vi "flow-builder.nutrition-sample.vi"(7 "Proc Name":string, 10 "Unit Index":i32) -> (0 "error out":errorcluster, 1 "status":string, 2 "Nutrition Will Dose?":bool, 3 "intructions out":variant[](array[variant]), 4 "Unit Enable?":bool)   [LabVIEW 2024]
uses:
  controls/UiStepBuilder.ctl
  controls/type.step-builder.ctl
  <vilib>/Utility/error.llb/Trim Whitespace.vi
  build.flowToVarient.vi
  <vilib>/Utility/error.llb/Trim Whitespace One-Sided.vi
  Polymorphics/variantCtrl.polymorphic.vi
  Polymorphics/variantCtrlStepFunction.vi
  Polymorphics/variantCtrlSetpoint.vi
  Polymorphics/variantCtrlString.vi
  proc.util.enumToStrStepVar.vi
  Polymorphics/variantCtrlNumber.vi
  util.DelimitedStringToArray.vi
  proc.util.validateParamExist.vi
  globals/globals-engine.vi
  build.elementToParamString.vi
  util.error.create.vi
  Polymorphics/variantCtrlStepPointer.vi
  Polymorphics/variantCtrlStepUserMessage.vi
  Polymorphics/variantCtrlStepPath.vi
panel:
  out "water Will Dose?":bool
  out "Flow":T1[](array[typedef])
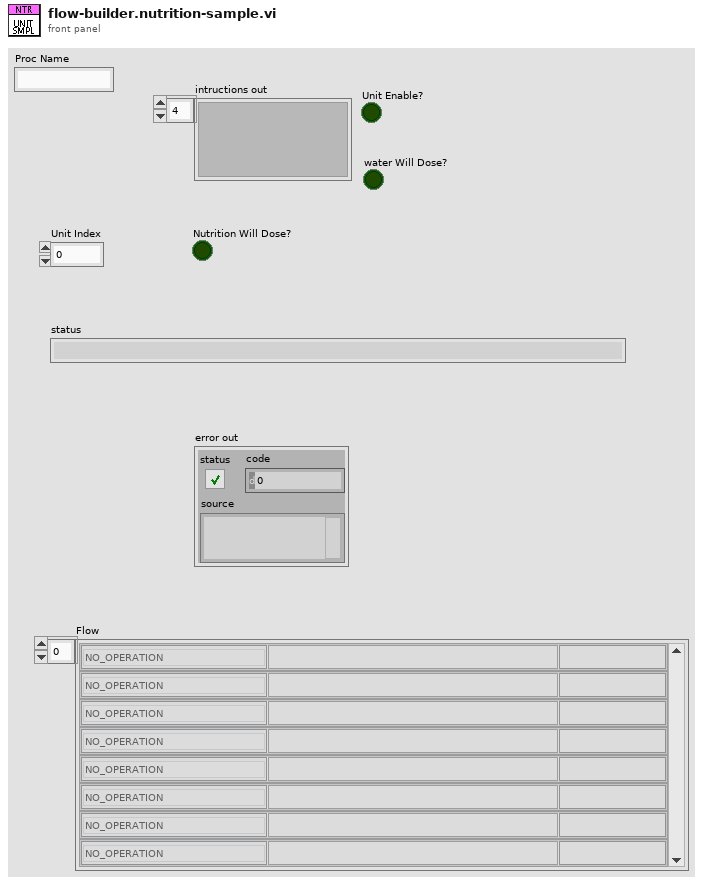
[diagram p1: front panel]
types:
  T1 = typedef "UiStepBuilder.ctl" = cluster{"Step Function":T2, "ParamString":string, "Step Label":string}
  T2 = typedef "type.step-builder.ctl" = enum16{"NO_OPERATION", "DELAY-JUMP", "DELAY", "JUMP", "COMPLETE", "SCHEDULER", "IRR-CHECK", "UNIT-CHECK", "UNIT-SAMPLE", "UNIT-DOSE", "LOG-REPORT", "LOG-MESSAGE", "IO-READ", "IO-READ-MANY", "IO-WRITE", "IO-COMPARE-OUT", "IO-COMPARE-IN", "PROC-START", "PROC-STOP", "PROC-LOAD", "PROC-IS-COMPLETED", "RECORD-MOVE", "GET-RH", "GET-UV", "GET-WD", "GET-WS", "OCS-CHECK", "OCS-RECORD"}
  T3 = typedef "UiNutritionPanel.ctl" = cluster{"Main":cluster{"Enable":bool, "WashTimes":cluster{"In":dbl, "Out":dbl}, "DailyActivityHours":cluster{"Begin Time":T4, "End Time":T4}[]}, "Water Dosing":cluster{"Water Dose":dbl, "Water Limit":dbl}, "EC Ranges":cluster{"H Alarm":dbl, "L Alarm":dbl, "Low":dbl}, "EC Dosing":cluster{"ALFA1 Dose":dbl, "ALFA1 Limit":dbl, "BETA1 Dose":dbl, "BETA1 Limit":dbl, "ALFA2 Dose":dbl, "ALFA2 Limit":dbl, "BETA2 Dose":dbl, "BETA2 Limit":dbl}, "PH Ranges":cluster{"H Alarm":dbl, "L Alarm":dbl, "High":dbl, "Low":dbl}, "PH Dosing":cluster{"ACID Dose":dbl, "ACID Limit":dbl, "BASE Dose":dbl, "BASE Limit":dbl}, "ORP Ranges":cluster{"H Alarm":dbl, "L Alarm":dbl, "Low":dbl}, "ORP Dosing":cluster{"MIX Dose":dbl, "MIX Limit":dbl}}
  T4 = typedef "UiScheduleTimestamp.ctl" = timestamp
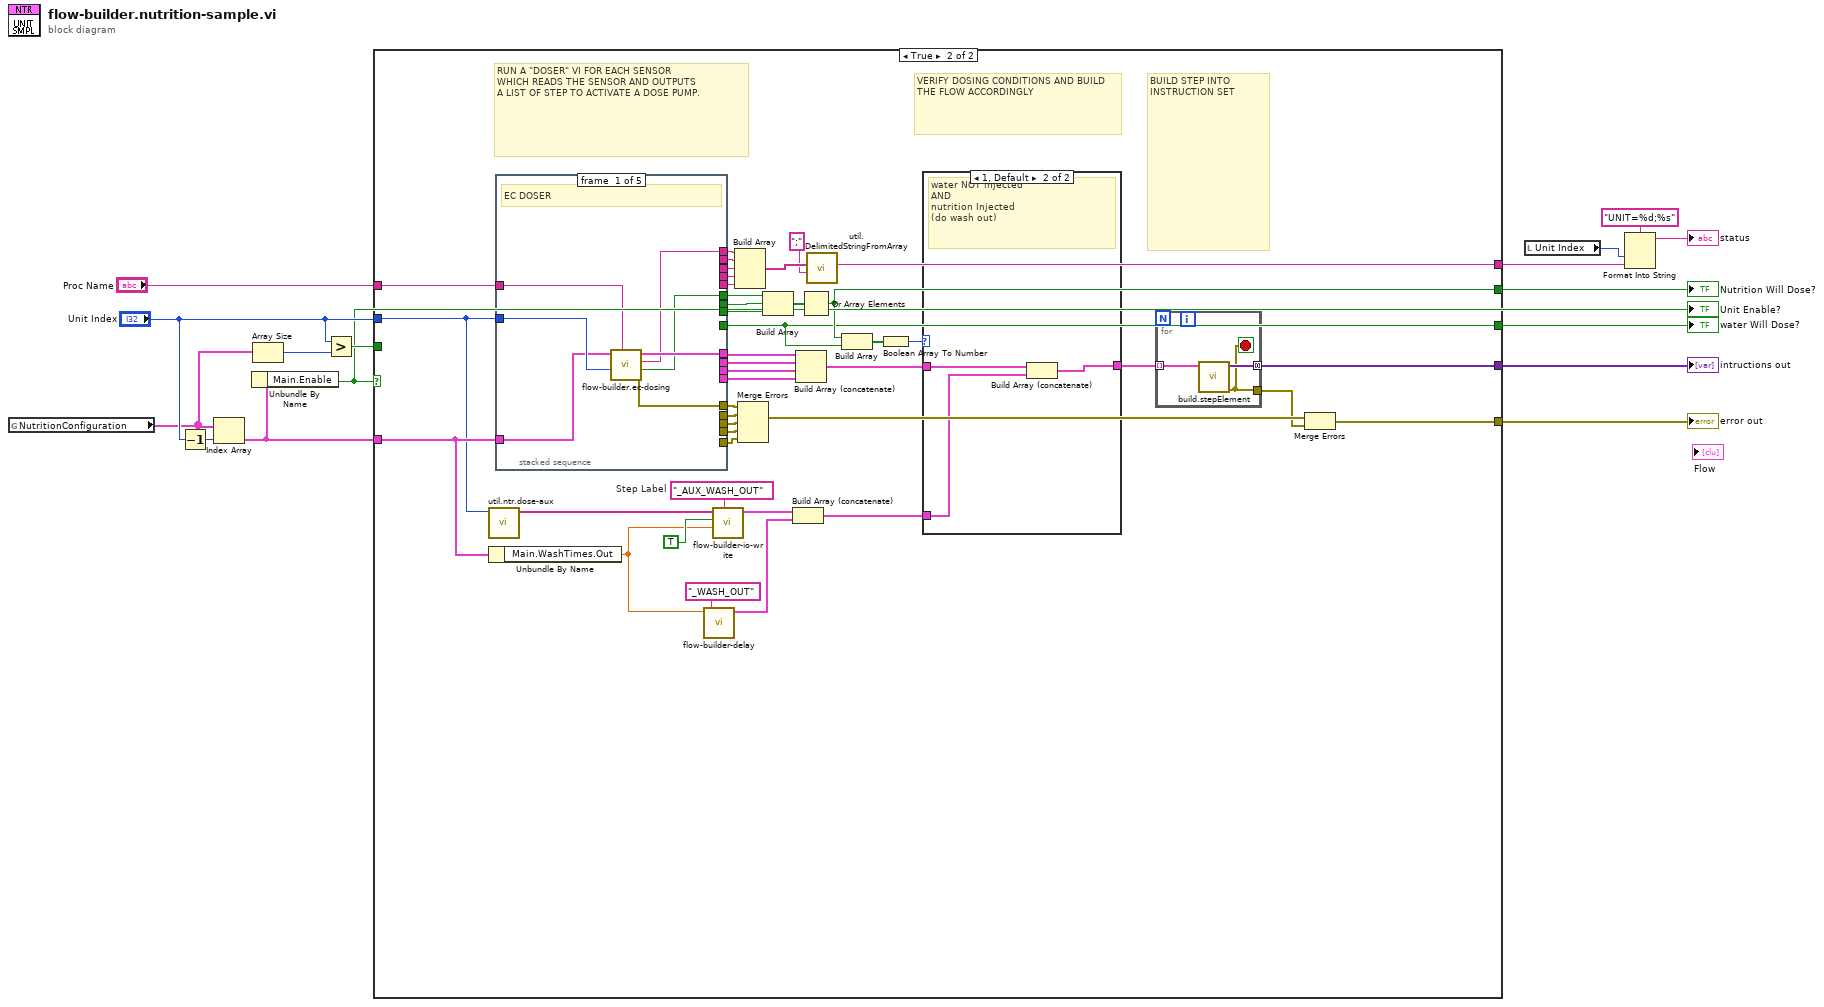
[diagram p0: block diagram]
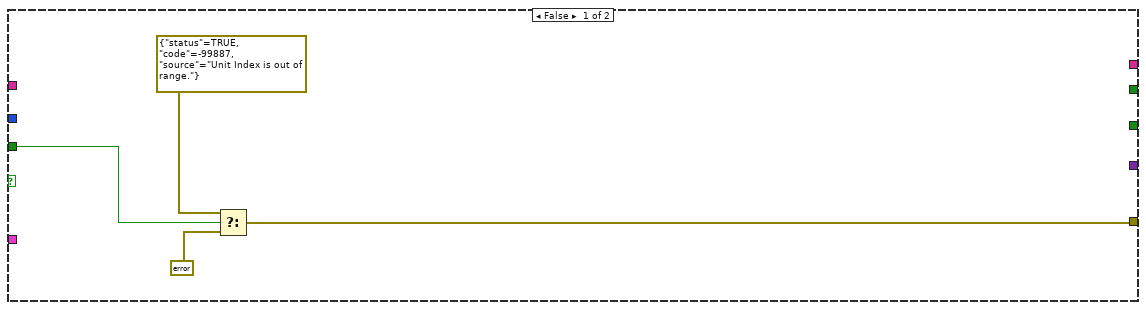
[diagram p2: hidden frame]
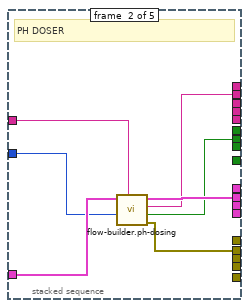
[diagram p4: hidden frame]
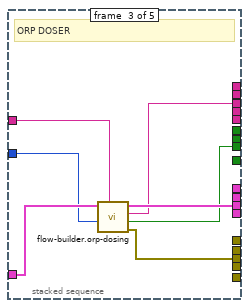
[diagram p5: hidden frame]
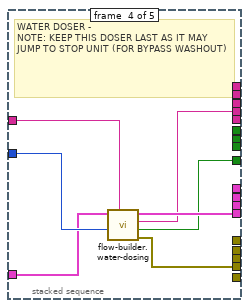
[diagram p6: hidden frame]
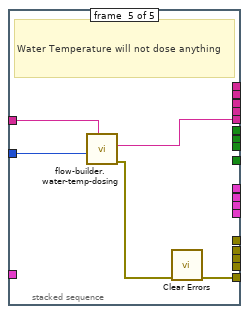
[diagram p7: hidden frame]
diagram:
  n1 = global read "globals-engine.vi" "NutritionConfiguration"() -> (w1:T3[])
  n2 = Decrement(x="Unit Index") -> (x-1=w14:i32)
  n3 = Index Array(array=w1, index=w14) -> (element=w13:T3)
  n4 = Unbundle By Name(w13) -> ("Main.Enable"=w4:bool)
  "Unit Enable?" <- w4
  n5 = Array Size(array=w1) -> (size(s)=w12:i32)
  n6 = Greater?(x="Unit Index", y=w12) -> (0:w11:bool)
  n7 = case shown="True" w4 {
    tunnel: [_ w35] -> w5
    tunnel: [_ w62] -> w16
    tunnel: [w18 w53] -> w15
    tunnel: "Unit Index" -> [_ w32]
    tunnel: w13 -> [_ w34]
    tunnel: w11 -> [w17 _]
    tunnel: [_ w49] -> w10
    tunnel: "Proc Name" -> [_ w33]
    tunnel: [_ w23] -> w3
    frame False {
      n8 = Select(t=errorcluster {"status"=TRUE, "code"=-99887, "source"="Unit Index is out of range."} ("error IO"), s=w17, f=errorcluster {"status"=FALSE, "code"=0, "source"=""} ("error IO")) -> (s? t:f=w18:errorcluster)
    }
    frame True {
      w26 = "_AUX_WASH_OUT"  # Step Label
      # "BUILD STEP INTO INSTRUCTION SET"
      # "VERIFY DOSING CONDITIONS AND BUILD THE FLOW ACCORDINGLY"
      # "RUN A \"DOSER\" VI FOR EACH SENSOR\nWHICH READS THE SENSOR AND OUTPUTS\nA LIST OF STEP TO ACTIVATE A DOSE PUMP."
      n9 = call "util.ntr.dose-aux.vi"("Unit Index"=w32) -> ("DO Unit Pumps"=w31:string[])  [unwired: 6 in, 4 out]
      n10 = Unbundle By Name(w34) -> ("Main.WashTimes.Out"=w24:dbl)
      n11 = stacked-sequence {
        tunnel: [_ w83 _ _ _] -> w61
        tunnel: [w76 _ _ _ _] -> w44
        tunnel: [w75 _ _ _ _] -> w60
        tunnel: [w74 _ _ _ _] -> w59
        tunnel: [_ w82 _ _ _] -> w58
        tunnel: [_ w81 _ _ _] -> w57
        tunnel: w34 -> [w72 w80 w90 w92 _]
        tunnel: [_ _ _ w93 _] -> w56
        tunnel: [_ _ w89 _ _] -> w45
        tunnel: [_ _ w84 _ _] -> w55
        tunnel: w32 -> [w73 w78 w87 w95 w101]
        tunnel: [_ _ _ w94 _] -> w48
        tunnel: [_ _ w88 _ _] -> w47
        tunnel: w33 -> [w71 w79 w86 w97 w98]
        tunnel: [_ _ _ w96 _] -> w46
        tunnel: [w70 _ _ _ _] -> w42
        tunnel: [_ _ _ w91 _] -> w23
        tunnel: [_ w77 _ _ _] -> w41
        tunnel: [_ _ w85 _ _] -> w40
        tunnel: [_ _ _ _ w102] -> w22
        tunnel: [_ _ _ _ w99] -> w21
        frame #0 {
          # "EC DOSER"
          n12 = call "flow-builder.ec-dosing.vi"("Proc Name"=w71, "Unit Index"=w73, "Cluster"=w72) -> ("error out"=w74:errorcluster, "WillDose?"=w70:bool, "status"=w75:string, "Flow out"=w76:T1[])  [unwired: 5 in]
        }
        frame #1 {
          # "PH DOSER"
          n13 = call "flow-builder.ph-dosing.vi"("Proc Name"=w79, "Unit Index"=w78, "Cluster"=w80) -> ("error out"=w82:errorcluster, "WillDose?"=w77:bool, "status"=w81:string, "Flow out"=w83:T1[])  [unwired: 5 in]
        }
        frame #2 {
          # "ORP DOSER"
          n14 = call "flow-builder.orp-dosing.vi"("Proc Name"=w86, "Unit Index"=w87, "Nutrition Cluster"=w90) -> ("error out"=w84:errorcluster, "WillDose?"=w85:bool, "status"=w88:string, "Flow out"=w89:T1[])  [unwired: 5 in]
        }
        frame #3 {
          # "WATER DOSER - \nNOTE: KEEP THIS DOSER LAST AS IT MAY JUMP TO STOP UNIT (FOR BYPASS WASHOUT)"
          n15 = call "flow-builder.water-dosing.vi"("Proc Name"=w97, "Unit Index"=w95, "Cluster"=w92) -> ("error out"=w94:errorcluster, "Not Limited?"=w91:bool, "status"=w93:string, "Flow out"=w96:T1[])  [unwired: 5 in]
        }
        frame #4 {
          # "Water Temperature will not dose anything"
          n16 = call "flow-builder.water-temp-dosing.vi"("Proc Name"=w98, "Unit Index"=w101) -> ("error out"=w100:errorcluster, "status"=w102:string)  [unwired: 6 in, 2 out]
          n17 = call <vilib>:"Clear Errors.vi"("error in (no error)"=w100) -> ("error out"=w99:errorcluster)  [unwired: 5 in, 1 out]
        }
      }
      n18 = call "flow-builder-delay.vi"("Step Label"="_WASH_OUT", "Delay [s]"=w24) -> ("Step Element"=w28:T1)  [unwired: 9 in]
      n19 = call "flow-builder-io-write.vi"("Step Name"=w26, "Digital Timeout"=w24, "Value in"=TRUE ("UiDeviceConstant"), "Dout+AUX"=w31) -> ("Flow out"=w29:T1[])  [unwired: 7 in]
      n20 = Build Array(w60, w57, w47, w56, w22) -> (w51:string[])
      n21 = Merge Errors(w59, w58, w55, w48, w21) -> (w54:errorcluster)
      n22 = Build Array(w42, w41, w40) -> (w43:bool[])
      n23 = Build Array (concatenate)(w29, w28) -> (w30:T1[])
      n24 = Build Array (concatenate)(w44, w61, w45, w46) -> (w37:T1[])
      n25 = Or Array Elements(Boolean array=w43) -> (logical OR=w35:bool)
      n26 = call "util.DelimitedStringFromArray.vi"("delimiter (Comma)"=";" ("delimiter (Tab)"), "params array in"=w51) -> ("delimited string out"=w49:string)  [unwired: 9 in]
      n27 = Build Array(w35, w23) -> (w39:bool[])
      n28 = Boolean Array To Number(Boolean array=w39) -> (number=w38:u32)
      n29 = case shown="1, Default" w38 {
        tunnel: [w63 w65] -> w36
        tunnel: w37 -> [w63 w66]
        tunnel: w30 -> [_ w64]
        frame 0, 2, 3 {
          # "assume next step is\nstop unit"
          # "water injected\nby pass washout (10,11) OR nothing injected"
        }
        frame 1, Default {
          # "water NOT injected\nAND\nnutrition Injected\n(do wash out)"
          n30 = Build Array (concatenate)(w66, w64) -> (w65:T1[])
        }
      }
      n31 = for {
        tunnel: w36 -> [w69] mode=indexing
        tunnel: [w68] -> w62 mode=concatenating
        tunnel: [w67] -> w52
        stop <- w67 stop-if-true
        n32 = call "build.stepElement.vi"("Step in"=w69) -> ("error out"=w67:errorcluster, "steps out"=w68:variant[])  [unwired: 9 in]
      }
      n33 = Merge Errors(w54, w52) -> (w53:errorcluster)
    }
  }
  "intructions out" <- w16
  "Nutrition Will Dose?" <- w5
  "error out" <- w15
  "water Will Dose?" <- w3
  n34 = local read "Unit Index"() -> (w2:i32)
  n35 = Format Into String(format string="UNIT=%d;%s", w2, w10) -> (resulting string=→"status":string)  [unwired: 2 in, 1 out]
